vi "RateScan_SINBUCLE.vi"() -> ()   [LabVIEW 2019]
uses:
  Viejos/Alfredo LABVIEW/Set-up verificador ASICs/Lib Agilent 81160A/Agilent 81150/Agilent 81150.lvlib
panel:
  out "Reg 101-100":u32 format="%x"
  out "error out":errorcluster
  out "HANDLE":u32
  out "Error (\"1\" Error)":bool
  out "Todos":T1(array[cluster])=[{"Device Index"=0, "FT_FLAGS_OPENED"=TRUE, "FT_FLAGS_HISPEED"=TRUE, "Type"=6, "VID"=1027, "PID"=24592, "LocID"=1131585, "Serial Number"="CTAV2022A", "Description"="MI CTA TEST A", "FT_Handle"=433820616}, {"Device Index"=1, "FT_FLAGS_OPENED"=TRUE, "FT_FLAGS_HISPEED"=TRUE, "Type"=6, "VID"=1027, "PID"=24592, "LocID"=1131586, "Serial Number"="CTAV2022B", "Description"="MI CTA TEST B", "FT_Handle"=433822896}]
  out "Array CTA":T1(array[cluster])=[{"Device Index"=0, "FT_FLAGS_OPENED"=TRUE, "FT_FLAGS_HISPEED"=TRUE, "Type"=6, "VID"=1027, "PID"=24592, "LocID"=1131585, "Serial Number"="CTAV2022A", "Description"="MI CTA TEST A", "FT_Handle"=433820616}]
  out "DAC TH3,TH4,TH5":u16
  out "LLTHx":dbl
  out "DAC TH0,TH1,TH2":u16
  out "HLTHx":dbl
  out "x*y":u32 format="%x"
  out "Valor Asic default":u16 format="%x"
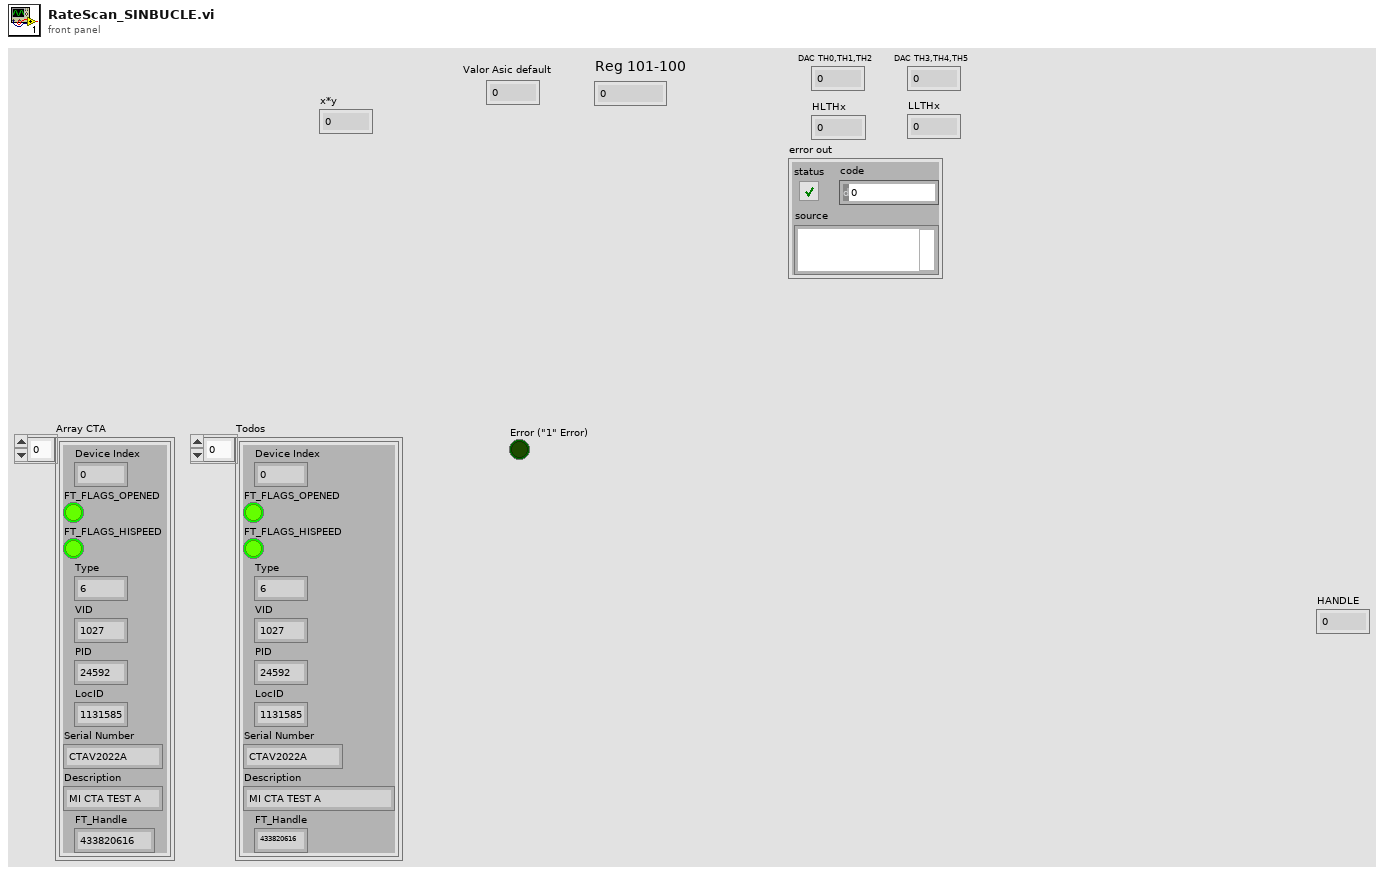
[diagram p1: front panel]
types:
  T1 = cluster{"Device Index":u32, "FT_FLAGS_OPENED":bool, "FT_FLAGS_HISPEED":bool, "Type":u32, "VID":u32, "PID":u32, "LocID":i32, "Serial Number":string, "Description":string, "FT_Handle":u32}[]
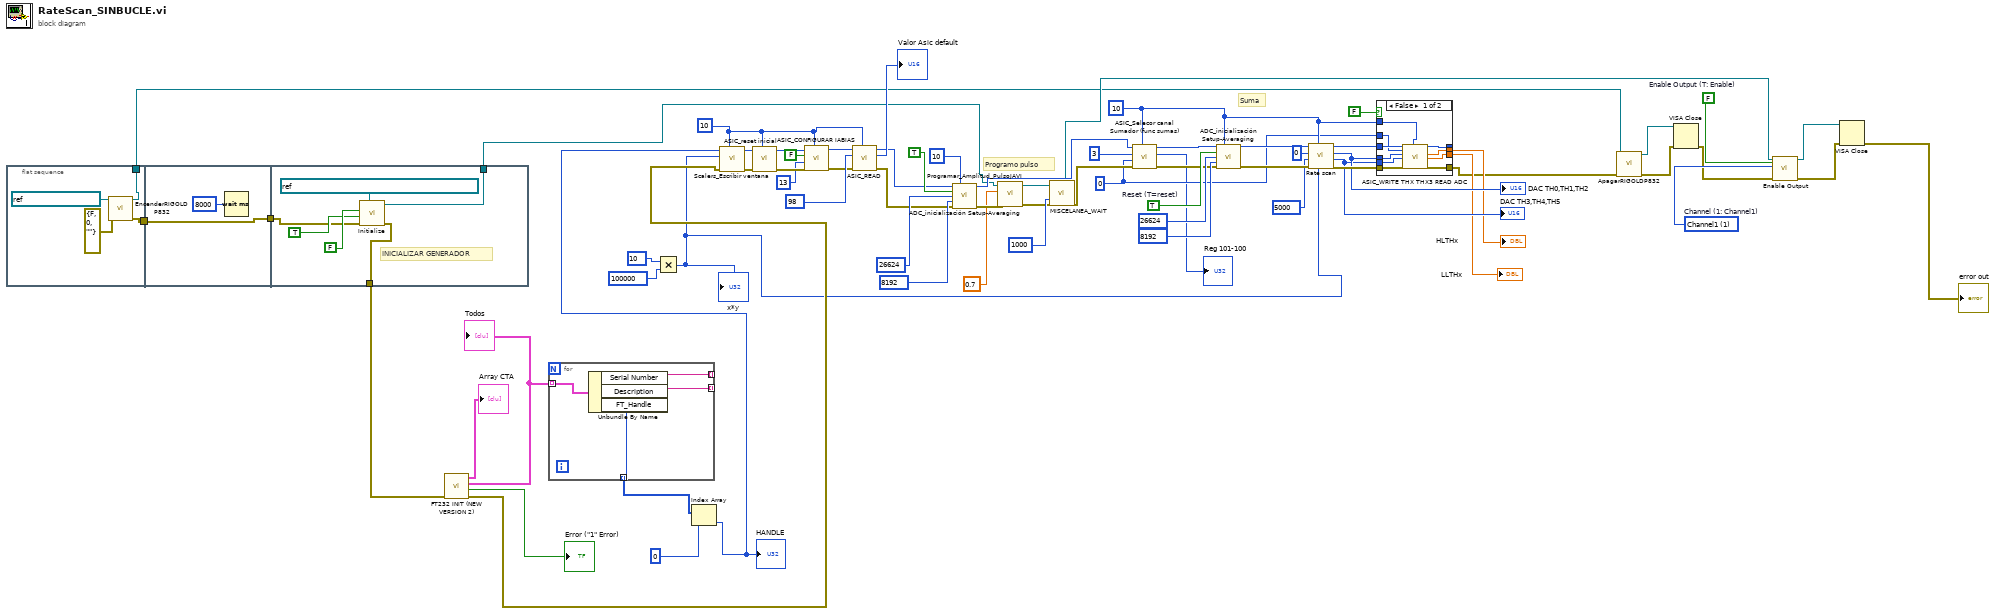
[diagram p0: block diagram]
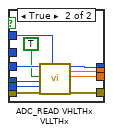
[diagram p2: hidden frame]
diagram:
  w27 = u16 1 items=["Channel1"=1, "Channel2"=2]  # Channel (1: Channel1)
  w28 = FALSE  # Enable Output (T: Enable)
  w10 = u8 0 ("Sumador")
  w44 = u32 10 ("Espera acceso USB")
  w55 = TRUE  # Reset (T=reset)
  w6 = u32 10 ("Espera acceso USB")
  # "Suma"
  # "Programo pulso"
  n1 = flat-sequence {
    tunnel: [w71] -> w17
    tunnel: [w70] -> w16
    tunnel: w16 -> [w74]
    tunnel: [w74] -> w15
    tunnel: w15 -> [w78]
    tunnel: [w77] -> w14
    tunnel: [w75] -> w13
    frame #0 {
      n2 = call "EncenderRIGOLDP832.vi"("error in (no error)"=errorcluster {"status"=FALSE, "code"=0, "source"=""}, "VISA IN"=refnum<visa-resource-name> "FA_Rigol_DP832") -> ("error out"=w70:errorcluster, "VISA resource name out"=w71:refnum<visa-resource-name>)  [unwired: 8 in]
    }
    frame #1 {
      n3 = Wait (ms)(milliseconds to wait=u32 8000) -> ()  [unwired: 1 out]
    }
    frame #2 {
      # "INICIALIZAR GENERADOR"
      n4 = call "Initialize.vi"("error in (no error)"=w78, "Reset (True)"=TRUE, "ID Query (True)"=FALSE, "VISA resource name"=refnum<visa-resource-name> "USB0::0x0957::0x4108::MY51400682::INSTR") -> ("error out"=w77:errorcluster, "VISA resource name out"=w75:refnum<visa-resource-name>)  [unwired: 6 in]
    }
  }
  n5 = call "FT232 INIT (NEW VERSION 2).vi"("error in (no error)"=w14) -> ("error out"=w26:errorcluster, "Error (\"1\" Error)"=→"Error (\"1\" Error)":bool, "Todos"=w37:T1, "Array CTA"=→"Array CTA":T1)  [unwired: 7 in]
  "Todos" <- w37
  n6 = for {
    tunnel: w37 -> [w84] mode=indexing
    tunnel: [w83] -> _ mode=indexing
    tunnel: [w82] -> _ mode=indexing
    tunnel: [w81] -> w38 mode=indexing
    n7 = Unbundle By Name(w84) -> ("Serial Number"=w83:string, "Description"=w82:string, "FT_Handle"=w81:u32)
  }
  n8 = Multiply(x=u32 10 ("Ventana"), y=u32 100000 ("Ventana")) -> (x*y=w9:u32)
  "x*y" <- w9
  n9 = Index Array(array=w38, index=0) -> (element=w31:u32)
  "HANDLE" <- w31
  n10 = call "Scalers_Escribir ventana.vi"("Espera acceso USB"=w6, "error in"=w26, "Ventana"=w9, "ftHandle_in"=w31) -> ("error out"=w68:errorcluster, "ftHandle_out"=w67:u32)  [unwired: 6 in]
  n11 = call "ASIC_reset inicial.vi"("Espera acceso USB"=w6, "error in"=w68, "ftHandle_in"=w67) -> ("error out"=w3:errorcluster, "ftHandle_out"=w7:u32)  [unwired: 7 in]
  n12 = call "ASIC_CONFIGURAR IABIAS.vi"("Espera acceso USB"=w6, "error in"=w3, "IBIAS VALUE"=u8 13, "IBIAS"=FALSE, "ftHandle_in"=w7) -> ("error out"=w5:errorcluster, "ftHandle_out"=w4:u32)  [unwired: 5 in]
  n13 = call "ASIC_READ.vi"("Espera acceso USB"=w6, "error in"=w5, "Direccion Registro Asic"=u8 98, "ftHandle_in"=w4) -> ("error out"=w32:errorcluster, "Valor Asic"=→"Valor Asic default":u16, "ftHandle_out"=w33:u32)  [unwired: 5 in]
  n14 = call "ADC_inicialización Setup-Averaging.vi"("ftHandle_in 2"=w33, "Espera acceso USB"=u32 10, "Reset (T=reset)"=TRUE, "Registro Setup (0x6800)"=u16 26624, "Registro Averaging (0x3200)"=u16 8192 ("Registro Setup (0x6800)"), "error in 2"=w32) -> ("ftHandle_out"=w30:u32, "error out"=w58:errorcluster)  [unwired: 8 in]
  n15 = call "Programar_Amplitud_PulsoJAVI.vi"("error in (no error)"=w58, "Numeric"=0.7, "VISA Refnum in"=w13) -> ("Error OUT"=w61:errorcluster, "VISA resource name out"=w25:refnum<visa-resource-name>)  [unwired: 7 in]
  n16 = call "MISCELANEA_WAIT.vi"("ms wait IN"=u32 1000, "Error IN"=w61) -> ("Error OUT"=w29:errorcluster)  [unwired: 16 in, 1 out]
  n17 = call "ASIC_Selecor canal Sumador (func sumas).vi"("Espera acceso USB"=w44, "error in"=w29, "Sumador"=w10, "Modo"=u8 3, "ftHandle_in"=w30) -> ("error out"=w50:errorcluster, "Reg 101-100"=→"Reg 101-100":u32, "ftHandle_out"=w47:u32)  [unwired: 3 in, 1 out]
  n18 = call "ADC_inicialización Setup-Averaging.vi"("ftHandle_in 2"=w47, "Espera acceso USB"=w44, "Reset (T=reset)"=w55, "Registro Setup (0x6800)"=u16 26624, "Registro Averaging (0x3200)"=u16 8192 ("Registro Setup (0x6800)"), "error in 2"=w50) -> ("ftHandle_out"=w52:u32, "error out"=w51:errorcluster)  [unwired: 8 in]
  n19 = call "Rate scan.vi"("T Ventana"=w9, "Espera acceso USB"=w44, "error in 2"=w51, "Valor buscado scalers (5000)"=u16 5000 ("Valor buscado scalers"), "Sumador"=u8 0, "ftHandle_in 2"=w52) -> ("error out 2"=w48:errorcluster, "DAC\nTH3,TH4,TH5"=w42:u16, "DAC\nTH0,TH1,TH2"=w43:u16, "ftHandle_out 2"=w49:u32)  [unwired: 1 in, 1 out]
  "DAC TH0,TH1,TH2" <- w43
  "DAC TH3,TH4,TH5" <- w42
  n20 = case shown="False" FALSE {
    tunnel: w49 -> [w94 w104]
    tunnel: w48 -> [w91 w103]
    tunnel: [w89 w102] -> _
    tunnel: [w90 w101] -> w24
    tunnel: [w88 w100] -> w41
    tunnel: [w87 w99] -> w40
    tunnel: w43 -> [w93 w98]
    tunnel: w42 -> [w92 w97]
    tunnel: w44 -> [w86 w95]
    tunnel: w10 -> [w85 _]
    frame False {
      n21 = call "ASIC_WRITE THX THX3 READ ADC.vi"("ftHandle_in"=w94, "Sumador"=w85, "THX"=w93, "THX+3"=w92, "error in"=w91, "Espera acceso USB 2"=w86) -> ("ftHandle_out"=w89:u32, "HLTHx"=w88:dbl, "LLTHx"=w87:dbl, "error out"=w90:errorcluster)  [unwired: 10 in]
    }
    frame True {
      n22 = call "ADC_READ VHLTHx VLLTHx.vi"("ftHandle_out 2"=w104, "referenciar"=TRUE, "ref DAC\nTH0,TH1,TH2"=w98, "ref DAC\nTH3,TH4,TH5"=w97, "error out 2"=w103, "Espera acceso FT"=w95) -> ("ftHandle_out"=w102:u32, "HLTHx"=w100:dbl, "LLTHx"=w99:dbl, "error out"=w101:errorcluster)  [unwired: 10 in]
    }
  }
  "HLTHx" <- w41
  "LLTHx" <- w40
  n23 = call "ApagarRIGOLDP832.vi"("error in (no error)"=w24, "VISA resource name"=w17) -> ("error out"=w22:errorcluster, "VISA resource name out"=w23:refnum<visa-resource-name>)  [unwired: 8 in]
  n24 = VISA Close(VISA resource name=w23, error in (no error)=w22) -> (error out=w21:errorcluster)
  n25 = call "Enable Output.vi"("Enable Output (T: Enable)"=w28, "error in (no error)"=w21, "Channel (1: Channel1)"=w27, "VISA resource name"=w25) -> ("error out"=w19:errorcluster, "VISA resource name out"=w20:refnum<visa-resource-name>)  [unwired: 6 in]
  n26 = VISA Close(VISA resource name=w20, error in (no error)=w19) -> (error out=→"error out":errorcluster)
